vi "Autonomous_Load.vi"(0 "Number of Commands":i32, 5 "Subsystems":string[](array[string]), 7 "Commands":string[](array[string]), 9 "Inputs":string[][](array[string]), 11 "error in":errorcluster) -> (4 "Queue_Key":refnum<queue>, 6 "Autonomous_Queue":refnum<queue>, 15 "errror out":errorcluster)   [LabVIEW 2019]
uses:
  Queue_Key_Data.ctl
  RobotSubsystemsCluster.ctl
  Subsystems/Drive/Drive_Cluster.ctl
  Subsystems/Drive/Drive_States.ctl
  Subsystems/Intake/Intake_Cluster.ctl
  Subsystems/Intake/Intake_States.ctl
  Subsystems/Magazine/Magazine_Cluster.ctl
  Subsystems/Magazine/Magazine_States.ctl
  Subsystems/Flywheel/Flywheel_Cluster.ctl
  Subsystems/Flywheel/Flywheel_States.ctl
  Subsystems/Turret/Turret_Cluster.ctl
  Subsystems/Turret/Turret_States.ctl
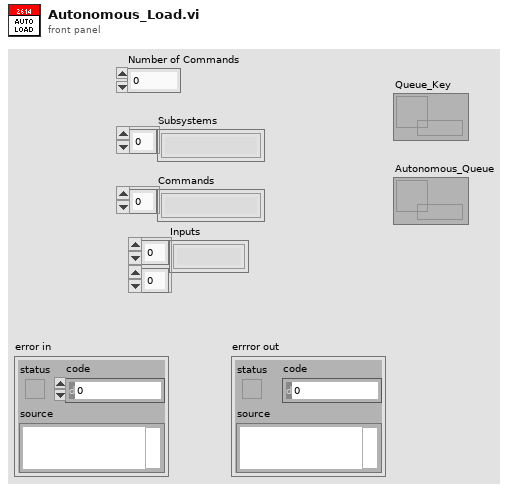
[diagram p1: front panel]
types:
  T1 = typedef "RobotSubsystemsCluster.ctl" = cluster{"Drive_Cluster":T2, "Intake_Cluster":T4, "Magazine_Cluster":T6, "Flywheel_Cluster":T8, "Turret_Cluster":T10}
  T2 = typedef "Drive_Cluster.ctl" = cluster{"Control_State":T3, "Angular_Throttle":dbl, "Linear_Throttle":dbl, "Torque_Changing":bool, "Step":dbl, "Parameter_1":dbl, "Parameter_2":dbl, "Parameter_3":dbl, "Parameter_4":dbl, "Auto_Notifier":refnum<notifier>}
  T3 = typedef "Drive_States.ctl" = enum16{"Percent_Voltage_Control", "Speed_Control"}
  T4 = typedef "Intake_Cluster.ctl" = cluster{"Control_State":T5, "Intake_On":bool, "Intake_Extended":bool, "Intake_Throttle":dbl, "Auto_Notifier":refnum<notifier>, "Parameter_1":dbl, "Parameter_2":dbl, "Step":dbl, "Outtake":bool}
  T5 = typedef "Intake_States.ctl" = enum16{"Manual_Control", "Compliant_Intake"}
  T6 = typedef "Magazine_Cluster.ctl" = cluster{"Fire":bool, "Magazine_Throttle":dbl, "Control_States":T7, "Auto_Notifier":refnum<notifier>, "Parameter_1":dbl, "Parameter_2":dbl, "Step":dbl}
  T7 = typedef "Magazine_States.ctl" = enum16{"No-Op", "Loading", "Fire", "Unjam", "Manual_Percent_Voltage", "Manual_Speed_Control"}
  T8 = typedef "Flywheel_Cluster.ctl" = cluster{"Flywheel_Throttle":dbl, "Control_States":T9, "Auto_Speed":bool, "Flywheel_On":bool, "Parameter_1":dbl, "Parameter_2":dbl, "Auto_Notifier":refnum<notifier>, "Step":dbl}
  T9 = typedef "Flywheel_States.ctl" = enum16{"No-Op", "Percent_Voltage", "Speed_Control_Manual", "Speed_Control_Auto"}
  T10 = typedef "Turret_Cluster.ctl" = cluster{"Auto-Target?":bool, "Control_State":T11, "Turret_Spin_Speed":dbl, "Turret_Spin_Speed_Control?":bool, "Step":dbl, "Parameter_1":dbl, "Parameter_2":dbl, "Parameter_3":dbl, "Auto_Notifier":refnum<notifier>}
  T11 = typedef "Turret_States.ctl" = enum16{"Manual_Percent_Voltage", "Manual_Speed_Control", "Auto-Target"}
  T12 = typedef "Queue_Key_Data.ctl" = cluster{"Operation Notifier":refnum<notifier>, "Subsystem":string, "Concurrent":bool}
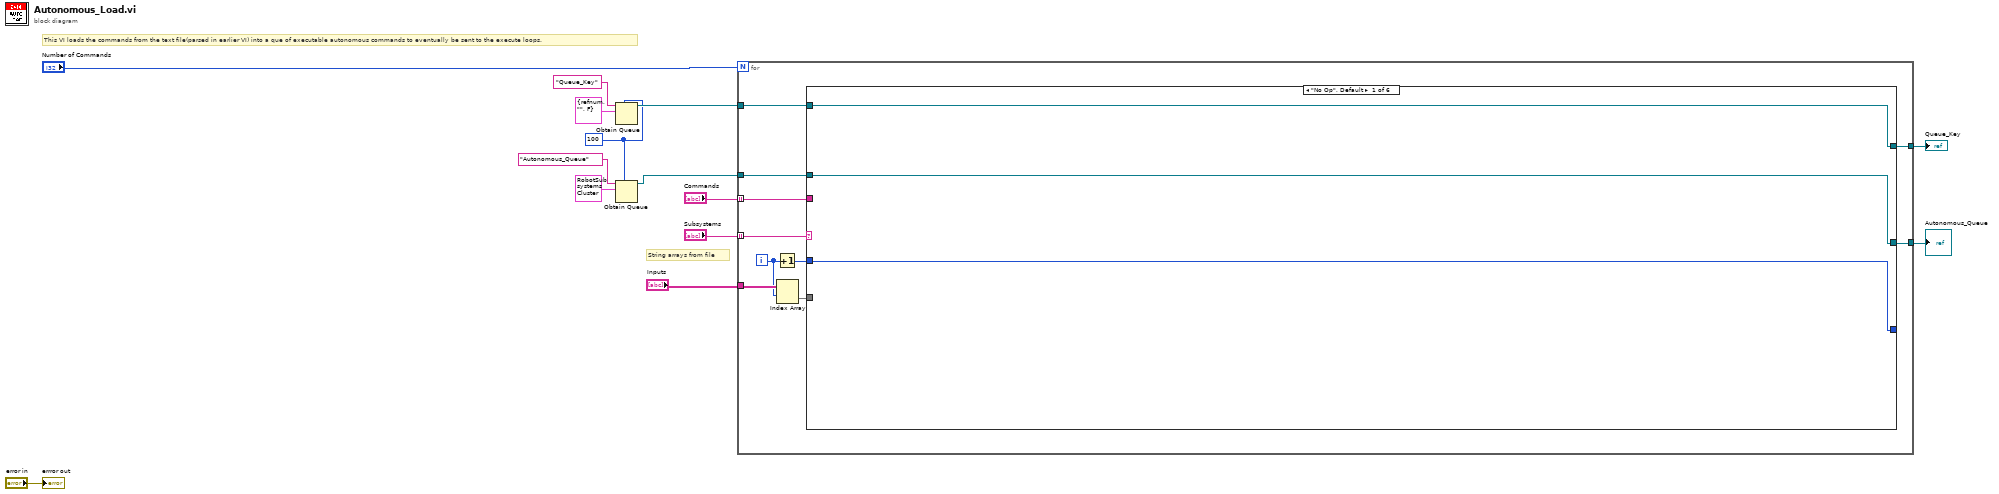
[diagram p0: block diagram]
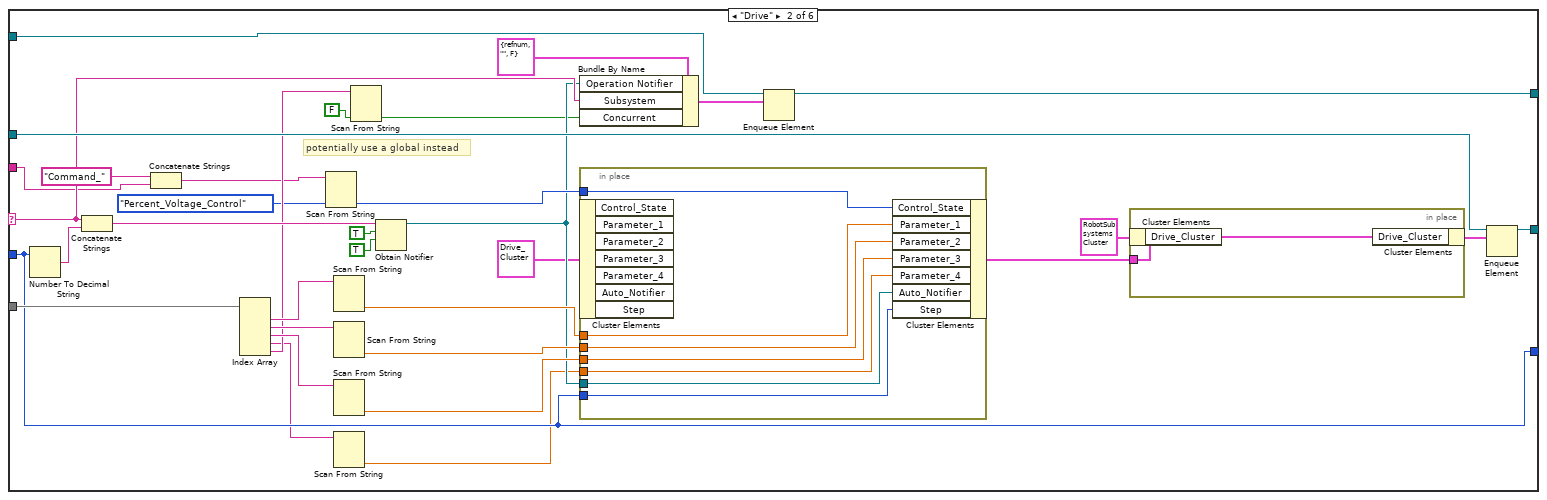
[diagram p2: hidden frame]
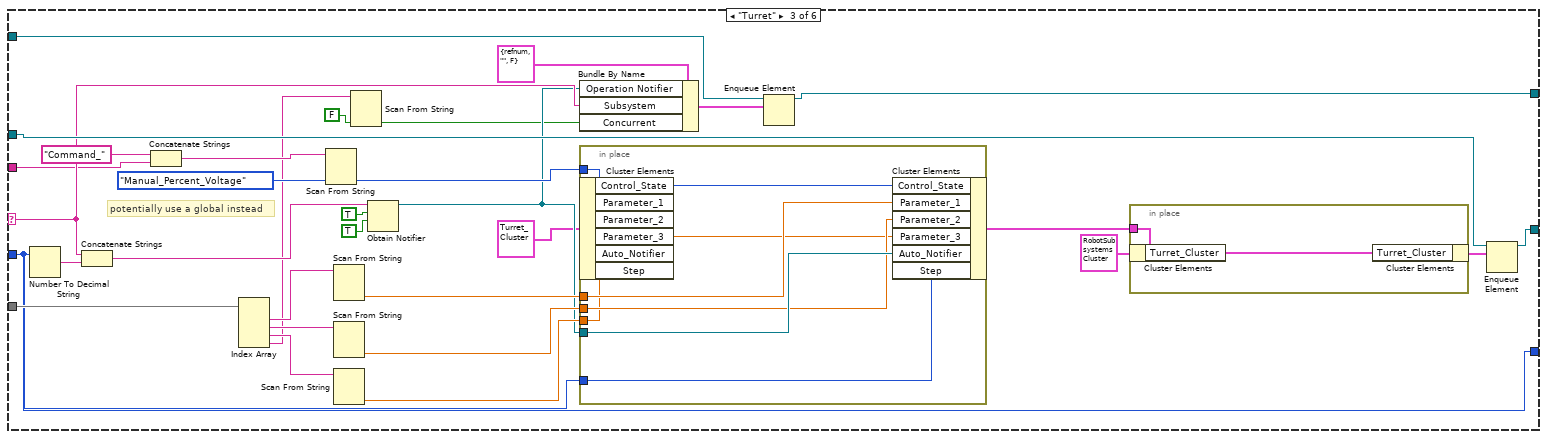
[diagram p3: hidden frame]
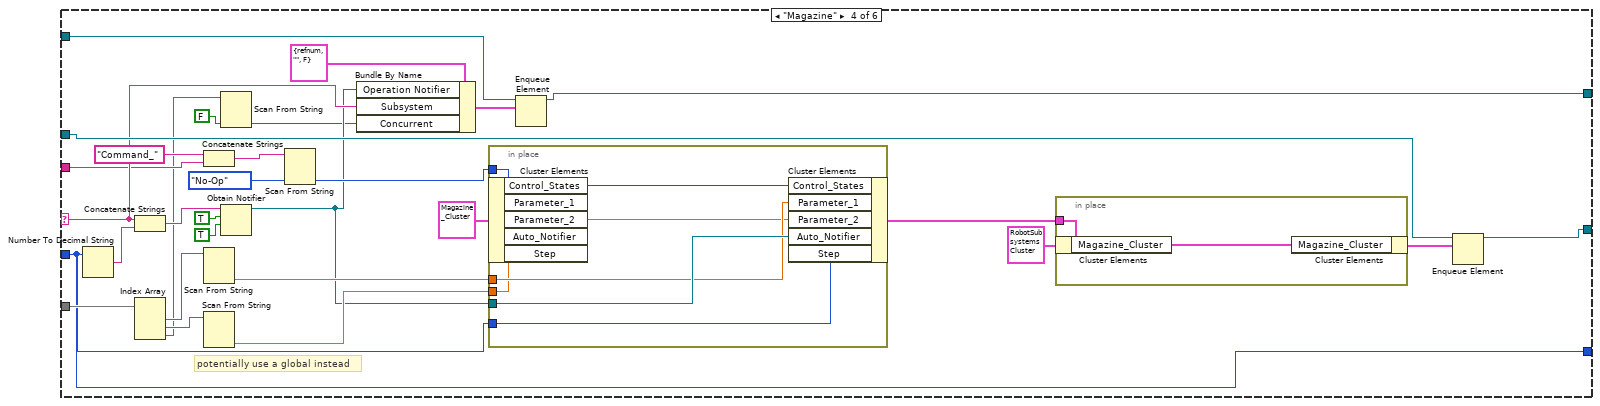
[diagram p4: hidden frame]
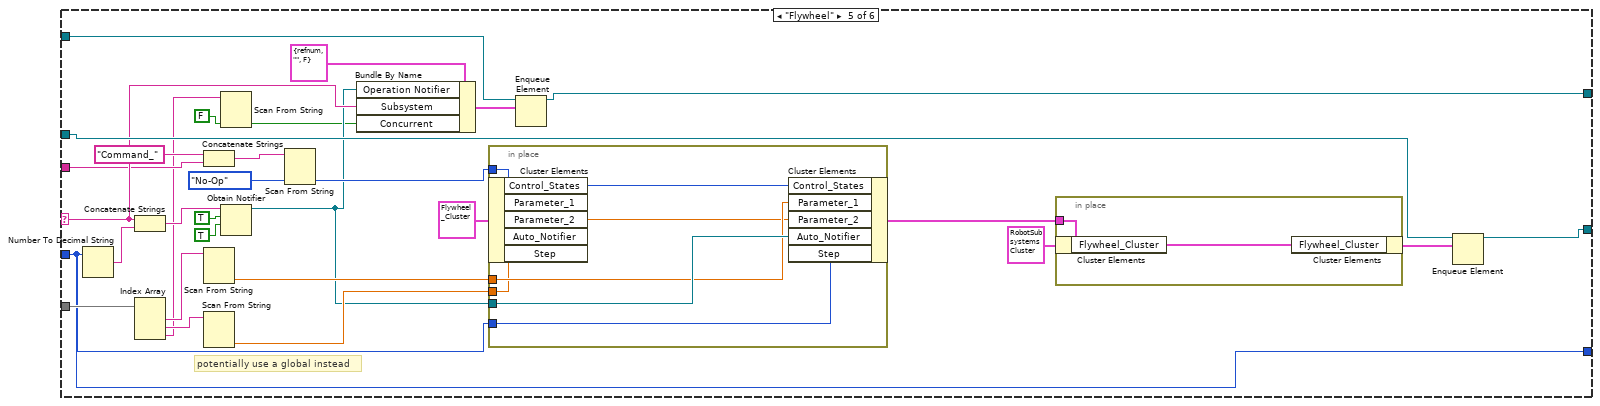
[diagram p5: hidden frame]
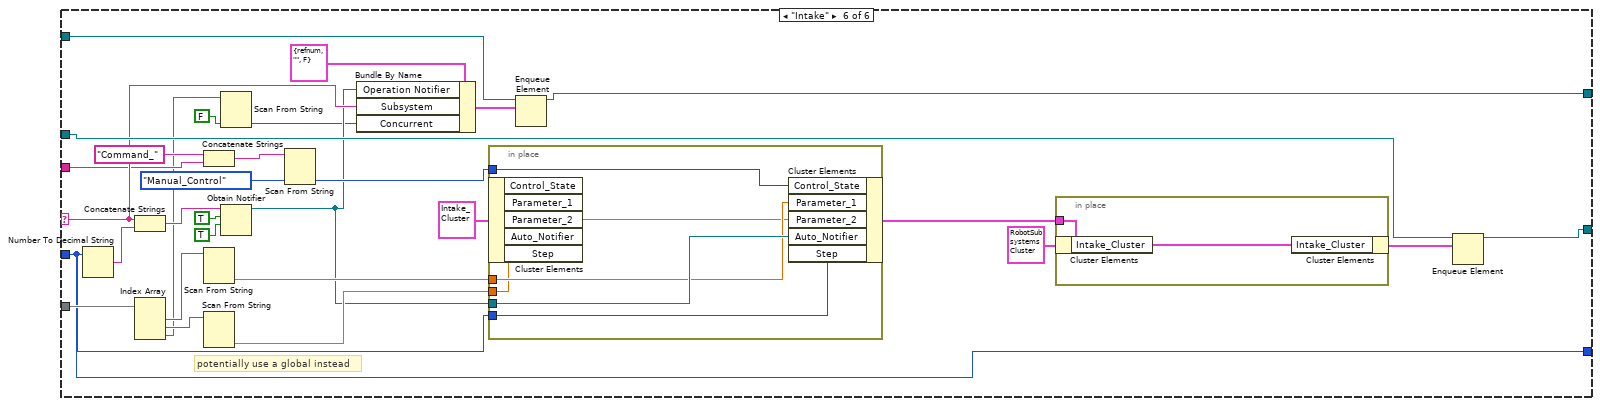
[diagram p6: hidden frame]
diagram:
  w6 = 100 ("max queue size (-1, unlimited)")
  # "This VI loads the commands from the text file(parsed in earlier VI) into a que of executable autonomous commands to eventually be sent to the execute loops."
  # "String arrays from file"
  n1 = Obtain Queue(max queue size (-1, unlimited)=w6, name (unnamed)="Queue_Key", element data type=T12 {"Operation Notifier"=refnum, "Subsystem"="", "Concurrent"=FALSE} ("Queue Key Data")) -> (queue out=w12:refnum<queue>)  [unwired: 2 in, 2 out]
  n2 = Obtain Queue(max queue size (-1, unlimited)=w6, name (unnamed)="Autonomous_Queue", element data type=T1 {"Drive_Cluster"={"Control_State"=enum."Percent_Voltage_Control", "Angular_Throttle"=0.0, "Linear_Throttle"=0.0, "Torque_Changing"=FALSE, "Step"=0.0, "Parameter_1"=0.0, "Parameter_2"=0.0, "Parameter_3"=0.0, "Parameter_4"=0.0, "Auto_Notifier"=refnum}, "Intake_Cluster"={"Control_State"=enum."Manual_Control", "Intake_On"=FALSE, "Intake_Extended"=FALSE, "Intake_Throttle"=0.0, "Auto_Notifier"=refnum, "Parameter_1"=0.0, "Parameter_2"=0.0, "Step"=0.0, "Outtake"=FALSE}, "Magazine_Cluster"={"Fire"=FALSE, "Magazine_Throttle"=0.0, "Control_States"=enum."No-Op", "Auto_Notifier"=refnum, "Parameter_1"=0.0, "Parameter_2"=0.0, "Step"=0.0}, "Flywheel_Cluster"={"Flywheel_Throttle"=0.0, "Control_States"=enum."No-Op", "Auto_Speed"=FALSE, "Flywheel_On"=FALSE, "Parameter_1"=0.0, "Parameter_2"=0.0, "Auto_Notifier"=refnum, "Step"=0.0}, "Turret_Cluster"={"Auto-Target?"=FALSE, "Control_State"=enum."Manual_Percent_Voltage", "Turret_Spin_Speed"=0.0, "Turret_Spin_Speed_Control?"=FALSE, "Step"=0.0, "Parameter_1"=0.0, "Parameter_2"=0.0, "Parameter_3"=0.0, "Auto_Notifier"=refnum}}) -> (queue out=w7:refnum<queue>)  [unwired: 2 in, 2 out]
  n3 = for {
    N: "Number of Commands" -> [_]
    tunnel: w12 -> [w24]
    tunnel: "Subsystems" -> [w23] mode=indexing
    tunnel: "Commands" -> [w22] mode=indexing
    tunnel: "Inputs" -> [w18]
    tunnel: [w21] -> w4
    tunnel: w7 -> [w20]
    tunnel: [w15] -> w1
    i -> [w16]
    n4 = Increment(x=w16) -> (x+1=w19:i32)
    n5 = Index Array(array=w18, index (row)=w16) -> (element=w17:string[])  [unwired: 1 in]
    n6 = case shown="\"No Op\", Default" w23 {
      selector: w23 -> [_ w41 w81 w120 w156 w192]
      tunnel: w24 -> [w26 w44 w84 w123 w159 w195]
      tunnel: w22 -> [_ w31 w74 w113 w149 w185]
      tunnel: [w27 w45 w85 w124 w160 w196] -> w15
      tunnel: [w26 w37 w77 w116 w152 w188] -> w21
      tunnel: w20 -> [w27 w48 w88 w127 w163 w199]
      tunnel: w19 -> [w25 w55 w95 w132 w168 w204]
      tunnel: [w25 w55 w95 w132 w168 w204] -> _
      tunnel: w17 -> [_ w56 w96 w133 w169 w205]
      frame "No Op", Default {
      }
      frame "Drive" {
        # "potentially use a global instead"
        n7 = Number To Decimal String(number=w55) -> (decimal integer string=w59:string)  [unwired: 1 in]
        n8 = Concatenate Strings(w41, w59) -> (w58:string)
        n9 = Concatenate Strings("Command_" ("string"), w31) -> (w32:string)
        n10 = Index Array(array=w56) -> (element #1=w54:string, element #2=w52:string, element #3=w49:string, element #4=w35:string, element #5=w36:string)  [unwired: 5 in]
        n11 = Scan From String(input string=w32, default 1=Drive_States."Percent_Voltage_Control" ("Control_State")) -> (output 1=w57:T3)  [unwired: 3 in, 3 out]
        n12 = Scan From String(input string=w54) -> (output 1=w53:dbl)  [unwired: 4 in, 3 out]
        n13 = Scan From String(input string=w52) -> (output 1=w51:dbl)  [unwired: 4 in, 3 out]
        n14 = Scan From String(input string=w49) -> (output 1=w50:dbl)  [unwired: 4 in, 3 out]
        n15 = Scan From String(input string=w35) -> (output 1=w34:dbl)  [unwired: 4 in, 3 out]
        n16 = Scan From String(input string=w36, default 1=FALSE) -> (output 1=w38:bool)  [unwired: 3 in, 3 out]
        n17 = Obtain Notifier(name (unnamed)=w58, notification data type=TRUE ("create if not found? (T)"), create if not found? (T)=TRUE) -> (notifier out=w40:refnum<notifier>)  [unwired: 1 in, 2 out]
        n18 = Bundle By Name(cluster=T12 {"Operation Notifier"=refnum, "Subsystem"="", "Concurrent"=FALSE} ("Queue Key Data"), "Operation Notifier"=w40, "Subsystem"=w41, "Concurrent"=w38) -> (w43:T12)
        n19 = in-place {
          in-place-border: w57 -> [w63]
          in-place-border: w40 -> [w69]
          in-place-border: w55 -> [w68]
          in-place-border: w53 -> [w67]
          in-place-border: w51 -> [w66]
          in-place-border: w50 -> [w65]
          in-place-border: w34 -> [w64]
          n20 = in-place-cluster #1(T2 {"Control_State"=enum."Percent_Voltage_Control", "Angular_Throttle"=0.0, "Linear_Throttle"=0.0, "Torque_Changing"=FALSE, "Step"=0.0, "Parameter_1"=0.0, "Parameter_2"=0.0, "Parameter_3"=0.0, "Parameter_4"=0.0, "Auto_Notifier"=refnum} ("Drive_Cluster")) -> ()  [unwired: 7 out]
          n21 = in-place-cluster #1("Control_State"=w63, "Parameter_1"=w67, "Parameter_2"=w66, "Parameter_3"=w65, "Parameter_4"=w64, "Auto_Notifier"=w69, "Step"=w68) -> (w47:T2)
        }
        n22 = Enqueue Element(queue=w44, element=w43) -> (queue out=w37:refnum<queue>)  [unwired: 2 in, 2 out]
        n23 = in-place {
          in-place-border: w47 -> [w62]
          n24 = in-place-cluster #2(T1 {"Drive_Cluster"={"Control_State"=enum."Percent_Voltage_Control", "Angular_Throttle"=0.0, "Linear_Throttle"=0.0, "Torque_Changing"=FALSE, "Step"=0.0, "Parameter_1"=0.0, "Parameter_2"=0.0, "Parameter_3"=0.0, "Parameter_4"=0.0, "Auto_Notifier"=refnum}, "Intake_Cluster"={"Control_State"=enum."Manual_Control", "Intake_On"=FALSE, "Intake_Extended"=FALSE, "Intake_Throttle"=0.0, "Auto_Notifier"=refnum, "Parameter_1"=0.0, "Parameter_2"=0.0, "Step"=0.0, "Outtake"=FALSE}, "Magazine_Cluster"={"Fire"=FALSE, "Magazine_Throttle"=0.0, "Control_States"=enum."No-Op", "Auto_Notifier"=refnum, "Parameter_1"=0.0, "Parameter_2"=0.0, "Step"=0.0}, "Flywheel_Cluster"={"Flywheel_Throttle"=0.0, "Control_States"=enum."No-Op", "Auto_Speed"=FALSE, "Flywheel_On"=FALSE, "Parameter_1"=0.0, "Parameter_2"=0.0, "Auto_Notifier"=refnum, "Step"=0.0}, "Turret_Cluster"={"Auto-Target?"=FALSE, "Control_State"=enum."Manual_Percent_Voltage", "Turret_Spin_Speed"=0.0, "Turret_Spin_Speed_Control?"=FALSE, "Step"=0.0, "Parameter_1"=0.0, "Parameter_2"=0.0, "Parameter_3"=0.0, "Auto_Notifier"=refnum}}) -> ()  [unwired: 1 out]
          n25 = in-place-cluster #2("Drive_Cluster"=w62) -> (w46:T1)
        }
        n26 = Enqueue Element(queue=w48, element=w46) -> (queue out=w45:refnum<queue>)  [unwired: 2 in, 2 out]
      }
      frame "Turret" {
        # "potentially use a global instead"
        n27 = Number To Decimal String(number=w95) -> (decimal integer string=w99:string)  [unwired: 1 in]
        n28 = Concatenate Strings(w81, w99) -> (w98:string)
        n29 = Concatenate Strings("Command_" ("string"), w74) -> (w75:string)
        n30 = Index Array(array=w96) -> (element #1=w94:string, element #2=w92:string, element #3=w89:string, element #4=w70:string)  [unwired: 4 in]
        n31 = Scan From String(input string=w75, default 1=Turret_States."Manual_Percent_Voltage" ("Control_State")) -> (output 1=w97:T11)  [unwired: 3 in, 3 out]
        n32 = Scan From String(input string=w94) -> (output 1=w93:dbl)  [unwired: 4 in, 3 out]
        n33 = Scan From String(input string=w92) -> (output 1=w91:dbl)  [unwired: 4 in, 3 out]
        n34 = Scan From String(input string=w89) -> (output 1=w90:dbl)  [unwired: 4 in, 3 out]
        n35 = Scan From String(input string=w70, default 1=FALSE) -> (output 1=w78:bool)  [unwired: 3 in, 3 out]
        n36 = Obtain Notifier(name (unnamed)=w98, notification data type=TRUE ("create if not found? (T)"), create if not found? (T)=TRUE) -> (notifier out=w80:refnum<notifier>)  [unwired: 1 in, 2 out]
        n37 = Bundle By Name(cluster=T12 {"Operation Notifier"=refnum, "Subsystem"="", "Concurrent"=FALSE} ("Queue Key Data"), "Operation Notifier"=w80, "Subsystem"=w81, "Concurrent"=w78) -> (w83:T12)
        n38 = in-place {
          in-place-border: w97 -> [w103]
          in-place-border: w80 -> [w108]
          in-place-border: w95 -> [w107]
          in-place-border: w93 -> [w106]
          in-place-border: w91 -> [w105]
          in-place-border: w90 -> [w104]
          n39 = in-place-cluster #3(T10 {"Auto-Target?"=FALSE, "Control_State"=enum."Manual_Percent_Voltage", "Turret_Spin_Speed"=0.0, "Turret_Spin_Speed_Control?"=FALSE, "Step"=0.0, "Parameter_1"=0.0, "Parameter_2"=0.0, "Parameter_3"=0.0, "Auto_Notifier"=refnum} ("Turret_Cluster")) -> ()  [unwired: 6 out]
          n40 = in-place-cluster #3("Control_State"=w103, "Parameter_1"=w106, "Parameter_2"=w105, "Parameter_3"=w104, "Auto_Notifier"=w108, "Step"=w107) -> (w87:T10)
        }
        n41 = Enqueue Element(queue=w84, element=w83) -> (queue out=w77:refnum<queue>)  [unwired: 2 in, 2 out]
        n42 = in-place {
          in-place-border: w87 -> [w102]
          n43 = in-place-cluster #4(T1 {"Drive_Cluster"={"Control_State"=enum."Percent_Voltage_Control", "Angular_Throttle"=0.0, "Linear_Throttle"=0.0, "Torque_Changing"=FALSE, "Step"=0.0, "Parameter_1"=0.0, "Parameter_2"=0.0, "Parameter_3"=0.0, "Parameter_4"=0.0, "Auto_Notifier"=refnum}, "Intake_Cluster"={"Control_State"=enum."Manual_Control", "Intake_On"=FALSE, "Intake_Extended"=FALSE, "Intake_Throttle"=0.0, "Auto_Notifier"=refnum, "Parameter_1"=0.0, "Parameter_2"=0.0, "Step"=0.0, "Outtake"=FALSE}, "Magazine_Cluster"={"Fire"=FALSE, "Magazine_Throttle"=0.0, "Control_States"=enum."No-Op", "Auto_Notifier"=refnum, "Parameter_1"=0.0, "Parameter_2"=0.0, "Step"=0.0}, "Flywheel_Cluster"={"Flywheel_Throttle"=0.0, "Control_States"=enum."No-Op", "Auto_Speed"=FALSE, "Flywheel_On"=FALSE, "Parameter_1"=0.0, "Parameter_2"=0.0, "Auto_Notifier"=refnum, "Step"=0.0}, "Turret_Cluster"={"Auto-Target?"=FALSE, "Control_State"=enum."Manual_Percent_Voltage", "Turret_Spin_Speed"=0.0, "Turret_Spin_Speed_Control?"=FALSE, "Step"=0.0, "Parameter_1"=0.0, "Parameter_2"=0.0, "Parameter_3"=0.0, "Auto_Notifier"=refnum}}) -> ()  [unwired: 1 out]
          n44 = in-place-cluster #4("Turret_Cluster"=w102) -> (w86:T1)
        }
        n45 = Enqueue Element(queue=w88, element=w86) -> (queue out=w85:refnum<queue>)  [unwired: 2 in, 2 out]
      }
      frame "Magazine" {
        # "potentially use a global instead"
        n46 = Number To Decimal String(number=w132) -> (decimal integer string=w136:string)  [unwired: 1 in]
        n47 = Concatenate Strings(w120, w136) -> (w135:string)
        n48 = Index Array(array=w133) -> (element #1=w131:string, element #2=w129:string, element #3=w109:string)  [unwired: 3 in]
        n49 = Concatenate Strings("Command_" ("string"), w113) -> (w114:string)
        n50 = Scan From String(input string=w131) -> (output 1=w130:dbl)  [unwired: 4 in, 3 out]
        n51 = Scan From String(input string=w129) -> (output 1=w128:dbl)  [unwired: 4 in, 3 out]
        n52 = Scan From String(input string=w109, default 1=FALSE) -> (output 1=w117:bool)  [unwired: 3 in, 3 out]
        n53 = Obtain Notifier(name (unnamed)=w135, notification data type=TRUE ("create if not found? (T)"), create if not found? (T)=TRUE) -> (notifier out=w119:refnum<notifier>)  [unwired: 1 in, 2 out]
        n54 = Scan From String(input string=w114, default 1=Magazine_States."No-Op" ("Control_States")) -> (output 1=w134:T7)  [unwired: 3 in, 3 out]
        n55 = Bundle By Name(cluster=T12 {"Operation Notifier"=refnum, "Subsystem"="", "Concurrent"=FALSE} ("Queue Key Data"), "Operation Notifier"=w119, "Subsystem"=w120, "Concurrent"=w117) -> (w122:T12)
        n56 = in-place {
          in-place-border: w134 -> [w140]
          in-place-border: w119 -> [w144]
          in-place-border: w132 -> [w143]
          in-place-border: w130 -> [w142]
          in-place-border: w128 -> [w141]
          n57 = in-place-cluster #5(T6 {"Fire"=FALSE, "Magazine_Throttle"=0.0, "Control_States"=enum."No-Op", "Auto_Notifier"=refnum, "Parameter_1"=0.0, "Parameter_2"=0.0, "Step"=0.0} ("Magazine_Cluster")) -> ()  [unwired: 5 out]
          n58 = in-place-cluster #5("Control_States"=w140, "Parameter_1"=w142, "Parameter_2"=w141, "Auto_Notifier"=w144, "Step"=w143) -> (w126:T6)
        }
        n59 = Enqueue Element(queue=w123, element=w122) -> (queue out=w116:refnum<queue>)  [unwired: 2 in, 2 out]
        n60 = in-place {
          in-place-border: w126 -> [w139]
          n61 = in-place-cluster #6(T1 {"Drive_Cluster"={"Control_State"=enum."Percent_Voltage_Control", "Angular_Throttle"=0.0, "Linear_Throttle"=0.0, "Torque_Changing"=FALSE, "Step"=0.0, "Parameter_1"=0.0, "Parameter_2"=0.0, "Parameter_3"=0.0, "Parameter_4"=0.0, "Auto_Notifier"=refnum}, "Intake_Cluster"={"Control_State"=enum."Manual_Control", "Intake_On"=FALSE, "Intake_Extended"=FALSE, "Intake_Throttle"=0.0, "Auto_Notifier"=refnum, "Parameter_1"=0.0, "Parameter_2"=0.0, "Step"=0.0, "Outtake"=FALSE}, "Magazine_Cluster"={"Fire"=FALSE, "Magazine_Throttle"=0.0, "Control_States"=enum."No-Op", "Auto_Notifier"=refnum, "Parameter_1"=0.0, "Parameter_2"=0.0, "Step"=0.0}, "Flywheel_Cluster"={"Flywheel_Throttle"=0.0, "Control_States"=enum."No-Op", "Auto_Speed"=FALSE, "Flywheel_On"=FALSE, "Parameter_1"=0.0, "Parameter_2"=0.0, "Auto_Notifier"=refnum, "Step"=0.0}, "Turret_Cluster"={"Auto-Target?"=FALSE, "Control_State"=enum."Manual_Percent_Voltage", "Turret_Spin_Speed"=0.0, "Turret_Spin_Speed_Control?"=FALSE, "Step"=0.0, "Parameter_1"=0.0, "Parameter_2"=0.0, "Parameter_3"=0.0, "Auto_Notifier"=refnum}}) -> ()  [unwired: 1 out]
          n62 = in-place-cluster #6("Magazine_Cluster"=w139) -> (w125:T1)
        }
        n63 = Enqueue Element(queue=w127, element=w125) -> (queue out=w124:refnum<queue>)  [unwired: 2 in, 2 out]
      }
      frame "Flywheel" {
        # "potentially use a global instead"
        n64 = Number To Decimal String(number=w168) -> (decimal integer string=w172:string)  [unwired: 1 in]
        n65 = Concatenate Strings(w156, w172) -> (w171:string)
        n66 = Index Array(array=w169) -> (element #1=w167:string, element #2=w165:string, element #3=w147:string)  [unwired: 3 in]
        n67 = Concatenate Strings("Command_" ("string"), w149) -> (w150:string)
        n68 = Scan From String(input string=w167) -> (output 1=w166:dbl)  [unwired: 4 in, 3 out]
        n69 = Scan From String(input string=w165) -> (output 1=w164:dbl)  [unwired: 4 in, 3 out]
        n70 = Scan From String(input string=w147, default 1=FALSE) -> (output 1=w153:bool)  [unwired: 3 in, 3 out]
        n71 = Obtain Notifier(name (unnamed)=w171, notification data type=TRUE ("create if not found? (T)"), create if not found? (T)=TRUE) -> (notifier out=w155:refnum<notifier>)  [unwired: 1 in, 2 out]
        n72 = Scan From String(input string=w150, default 1=Flywheel_States."No-Op" ("Control_States")) -> (output 1=w170:T9)  [unwired: 3 in, 3 out]
        n73 = Bundle By Name(cluster=T12 {"Operation Notifier"=refnum, "Subsystem"="", "Concurrent"=FALSE} ("Queue Key Data"), "Operation Notifier"=w155, "Subsystem"=w156, "Concurrent"=w153) -> (w158:T12)
        n74 = in-place {
          in-place-border: w170 -> [w176]
          in-place-border: w155 -> [w180]
          in-place-border: w168 -> [w179]
          in-place-border: w166 -> [w178]
          in-place-border: w164 -> [w177]
          n75 = in-place-cluster #7(T8 {"Flywheel_Throttle"=0.0, "Control_States"=enum."No-Op", "Auto_Speed"=FALSE, "Flywheel_On"=FALSE, "Parameter_1"=0.0, "Parameter_2"=0.0, "Auto_Notifier"=refnum, "Step"=0.0} ("Flywheel_Cluster")) -> ()  [unwired: 5 out]
          n76 = in-place-cluster #7("Control_States"=w176, "Parameter_1"=w178, "Parameter_2"=w177, "Auto_Notifier"=w180, "Step"=w179) -> (w162:T8)
        }
        n77 = Enqueue Element(queue=w159, element=w158) -> (queue out=w152:refnum<queue>)  [unwired: 2 in, 2 out]
        n78 = in-place {
          in-place-border: w162 -> [w175]
          n79 = in-place-cluster #8(T1 {"Drive_Cluster"={"Control_State"=enum."Percent_Voltage_Control", "Angular_Throttle"=0.0, "Linear_Throttle"=0.0, "Torque_Changing"=FALSE, "Step"=0.0, "Parameter_1"=0.0, "Parameter_2"=0.0, "Parameter_3"=0.0, "Parameter_4"=0.0, "Auto_Notifier"=refnum}, "Intake_Cluster"={"Control_State"=enum."Manual_Control", "Intake_On"=FALSE, "Intake_Extended"=FALSE, "Intake_Throttle"=0.0, "Auto_Notifier"=refnum, "Parameter_1"=0.0, "Parameter_2"=0.0, "Step"=0.0, "Outtake"=FALSE}, "Magazine_Cluster"={"Fire"=FALSE, "Magazine_Throttle"=0.0, "Control_States"=enum."No-Op", "Auto_Notifier"=refnum, "Parameter_1"=0.0, "Parameter_2"=0.0, "Step"=0.0}, "Flywheel_Cluster"={"Flywheel_Throttle"=0.0, "Control_States"=enum."No-Op", "Auto_Speed"=FALSE, "Flywheel_On"=FALSE, "Parameter_1"=0.0, "Parameter_2"=0.0, "Auto_Notifier"=refnum, "Step"=0.0}, "Turret_Cluster"={"Auto-Target?"=FALSE, "Control_State"=enum."Manual_Percent_Voltage", "Turret_Spin_Speed"=0.0, "Turret_Spin_Speed_Control?"=FALSE, "Step"=0.0, "Parameter_1"=0.0, "Parameter_2"=0.0, "Parameter_3"=0.0, "Auto_Notifier"=refnum}}) -> ()  [unwired: 1 out]
          n80 = in-place-cluster #8("Flywheel_Cluster"=w175) -> (w161:T1)
        }
        n81 = Enqueue Element(queue=w163, element=w161) -> (queue out=w160:refnum<queue>)  [unwired: 2 in, 2 out]
      }
      frame "Intake" {
        # "potentially use a global instead"
        n82 = Number To Decimal String(number=w204) -> (decimal integer string=w208:string)  [unwired: 1 in]
        n83 = Concatenate Strings(w192, w208) -> (w207:string)
        n84 = Index Array(array=w205) -> (element #1=w203:string, element #2=w201:string, element #3=w183:string)  [unwired: 3 in]
        n85 = Concatenate Strings("Command_" ("string"), w185) -> (w186:string)
        n86 = Scan From String(input string=w203) -> (output 1=w202:dbl)  [unwired: 4 in, 3 out]
        n87 = Scan From String(input string=w201) -> (output 1=w200:dbl)  [unwired: 4 in, 3 out]
        n88 = Scan From String(input string=w183, default 1=FALSE) -> (output 1=w189:bool)  [unwired: 3 in, 3 out]
        n89 = Obtain Notifier(name (unnamed)=w207, notification data type=TRUE ("create if not found? (T)"), create if not found? (T)=TRUE) -> (notifier out=w191:refnum<notifier>)  [unwired: 1 in, 2 out]
        n90 = Scan From String(input string=w186, default 1=Intake_States."Manual_Control" ("Control_State")) -> (output 1=w206:T5)  [unwired: 3 in, 3 out]
        n91 = Bundle By Name(cluster=T12 {"Operation Notifier"=refnum, "Subsystem"="", "Concurrent"=FALSE} ("Queue Key Data"), "Operation Notifier"=w191, "Subsystem"=w192, "Concurrent"=w189) -> (w194:T12)
        n92 = in-place {
          in-place-border: w206 -> [w212]
          in-place-border: w191 -> [w216]
          in-place-border: w204 -> [w215]
          in-place-border: w202 -> [w214]
          in-place-border: w200 -> [w213]
          n93 = in-place-cluster #9(T4 {"Control_State"=enum."Manual_Control", "Intake_On"=FALSE, "Intake_Extended"=FALSE, "Intake_Throttle"=0.0, "Auto_Notifier"=refnum, "Parameter_1"=0.0, "Parameter_2"=0.0, "Step"=0.0, "Outtake"=FALSE} ("Intake_Cluster")) -> ()  [unwired: 5 out]
          n94 = in-place-cluster #9("Control_State"=w212, "Parameter_1"=w214, "Parameter_2"=w213, "Auto_Notifier"=w216, "Step"=w215) -> (w198:T4)
        }
        n95 = Enqueue Element(queue=w195, element=w194) -> (queue out=w188:refnum<queue>)  [unwired: 2 in, 2 out]
        n96 = in-place {
          in-place-border: w198 -> [w211]
          n97 = in-place-cluster #10(T1 {"Drive_Cluster"={"Control_State"=enum."Percent_Voltage_Control", "Angular_Throttle"=0.0, "Linear_Throttle"=0.0, "Torque_Changing"=FALSE, "Step"=0.0, "Parameter_1"=0.0, "Parameter_2"=0.0, "Parameter_3"=0.0, "Parameter_4"=0.0, "Auto_Notifier"=refnum}, "Intake_Cluster"={"Control_State"=enum."Manual_Control", "Intake_On"=FALSE, "Intake_Extended"=FALSE, "Intake_Throttle"=0.0, "Auto_Notifier"=refnum, "Parameter_1"=0.0, "Parameter_2"=0.0, "Step"=0.0, "Outtake"=FALSE}, "Magazine_Cluster"={"Fire"=FALSE, "Magazine_Throttle"=0.0, "Control_States"=enum."No-Op", "Auto_Notifier"=refnum, "Parameter_1"=0.0, "Parameter_2"=0.0, "Step"=0.0}, "Flywheel_Cluster"={"Flywheel_Throttle"=0.0, "Control_States"=enum."No-Op", "Auto_Speed"=FALSE, "Flywheel_On"=FALSE, "Parameter_1"=0.0, "Parameter_2"=0.0, "Auto_Notifier"=refnum, "Step"=0.0}, "Turret_Cluster"={"Auto-Target?"=FALSE, "Control_State"=enum."Manual_Percent_Voltage", "Turret_Spin_Speed"=0.0, "Turret_Spin_Speed_Control?"=FALSE, "Step"=0.0, "Parameter_1"=0.0, "Parameter_2"=0.0, "Parameter_3"=0.0, "Auto_Notifier"=refnum}}) -> ()  [unwired: 1 out]
          n98 = in-place-cluster #10("Intake_Cluster"=w211) -> (w197:T1)
        }
        n99 = Enqueue Element(queue=w199, element=w197) -> (queue out=w196:refnum<queue>)  [unwired: 2 in, 2 out]
      }
    }
  }
  "Queue_Key" <- w4
  "Autonomous_Queue" <- w1
  "errror out" <- "error in"
